vi "main_GB.vi"() -> ()   [LabVIEW 2020]
panel:
  in  "Stop Button":bool
  in  "Setting Tab":enum32{"File", "Setting"}(tab)
  in  "file path (dialog if empty)":path=path "C:/Users/user/Desktop/AutoSampler/AutoSampler _GB/AutoSampler.txt"
  in  "start of read offset (chars.:0)":i32
  in  "max characters/row  (no limit:0)":i32
  out "mark after read (chars.)":i32=403
  in  "number of rows (all:-1)":i32=-1
  out "all rows":string[][](array[string])=[["58"], ["257"], ["0"], ["0"], ["58"], ["257"], ["130"], ["50"], ["58"], ["257"], ["0"], ["50"], ["58"], ["470"], ["0"], ["50"], ["58"], ["470"], ["185"], ["0"], ["58"], ["470"], ["0"], ["0"], ["120"], ["470"], ["0"], ["0"], ["120"], ["470"], ["195"], ["50"], ["120"], ["470"], ["0"], ["50"], ["120"], ["550"], ["0"], ["0"], ["120"], ["550"], ["195"], ["0"], ["120"], ["550"], ["0"], ["0"], ["120"], ["470"], ["0"], ["0"], ["120"], ["470"], ["195"], ["50"], ["120"], ["470"], ["0"], ["50"], ["120"], ["550"], ["0"], ["0"], ["120"], ["550"], ["195"], ["0"], ["120"], ["550"], ["0"], ["0"], ["120"], ["470"], ["0"], ["0"], ["120"], ["470"], ["195"], ["50"], ["120"], ["470"], ["0"], ["50"], ["120"], ["550"], ["0"], ["0"], ["120"], ["550"], ["195"], ["0"], ["120"], ["550"], ["0"], ["0"]]
  in  "format (%.3f)":string="%.3f"
  in  "transpose (no:F)":bool
  in  "type (empty)":string[][](array[string])
  in  "delimiter (Tab)":string="\t"
  out "EOF?":bool
  out "size(s)":i32=96
  in  "Reading Time(S)":dbl=5.0
  out "X, Y, Z, S":i32=3
  out "Index":i32=95
  out "element":string="0"
  out "double precision float":dbl
  out "Current Position(mm)":dbl
  out "Arrived":bool=TRUE
  in  "Occupied Length by Air(mm)":dbl format="%#_13g"
  out "error out":errorcluster={"status"=FALSE, "code"=1073676294, "source"="VISA Read in position_read.vi->main_GB.vi"}
  out "S Connecting":bool=TRUE
  out "Z Connecting":bool=TRUE
  out "Y Connecting":bool=TRUE
  out "X  Connecting":bool=TRUE
  in  "COM Port":refnum<visa-resource-name>="COM3"
  # "Position :"
  # "(set the Occupied length by Air if the target axis is syringe axis)"
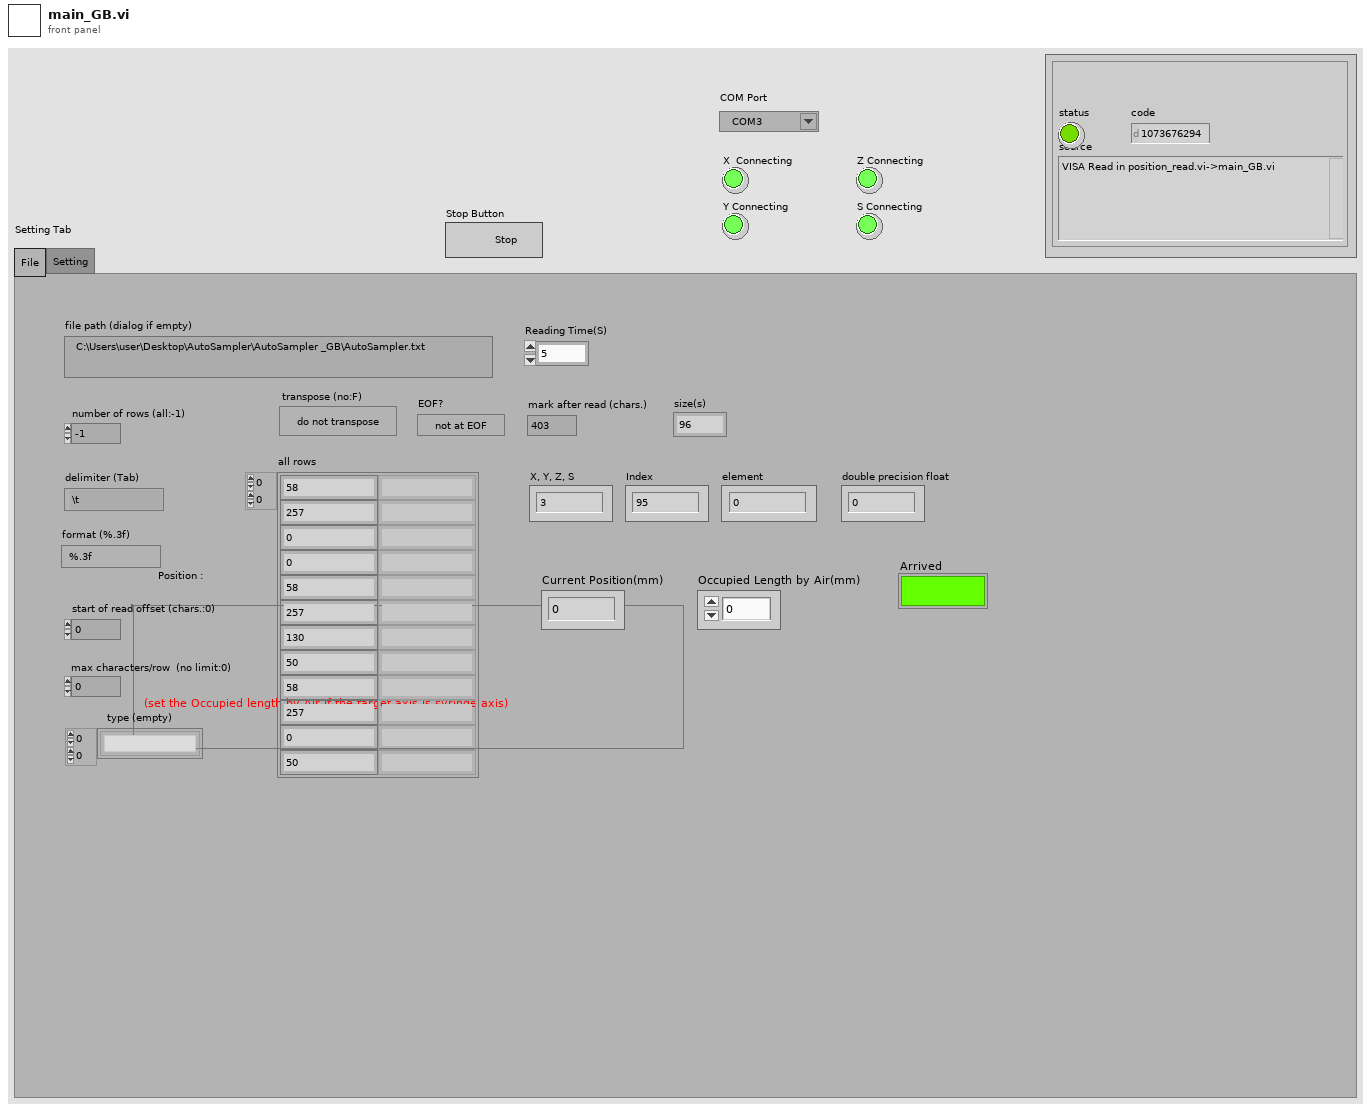
[diagram p1: front panel]
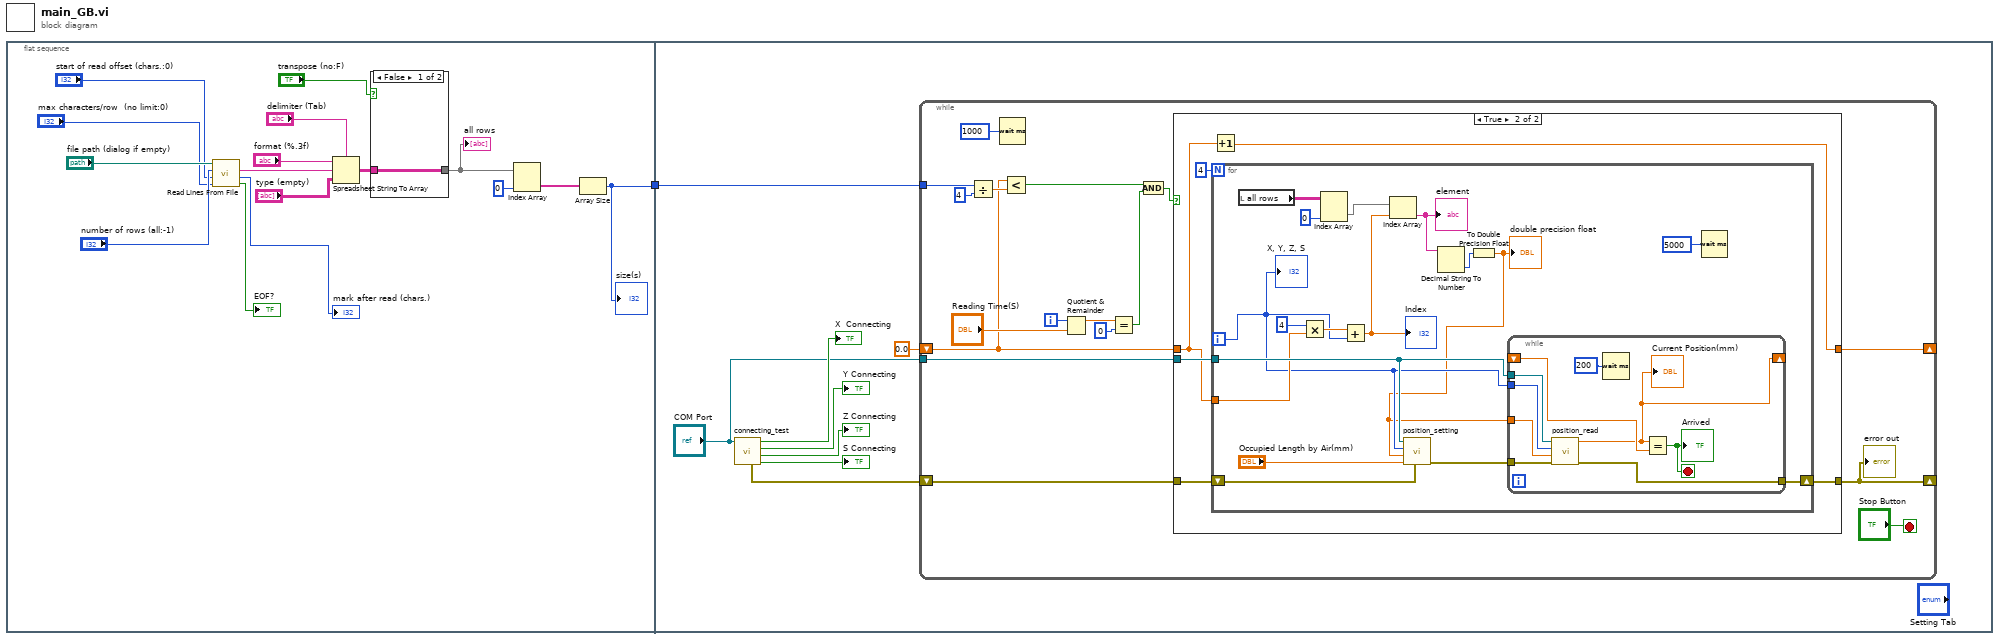
[diagram p0: block diagram]
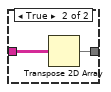
[diagram p2: hidden frame]
diagram:
  n1 = flat-sequence {
    tunnel: [w2] -> w1
    tunnel: w1 -> [w22]
    frame #0 {
      n2 = call <vilib>:"Read Lines From File.vi"("file path (dialog if empty)"="file path (dialog if empty)", "number of lines (all:-1)"="number of rows (all:-1)", "start of read offset (chars.:0)"="start of read offset (chars.:0)", "[max characters per line]  (no limit:0)"="max characters/row  (no limit:0)") -> ("line string"=w13:string, "mark after read (chars.)"=→"mark after read (chars.)":i32, "EOF?"=→"EOF?":bool)  [unwired: 2 in, 1 out]
      n3 = Spreadsheet String To Array(delimiter (Tab)="delimiter (Tab)", format string="format (%.3f)", spreadsheet string=w13, array type (2D Dbl)="type (empty)") -> (array=w11:string[][])
      n4 = case shown="False" "transpose (no:F)" {
        tunnel: [w18 w20] -> w5
        tunnel: w11 -> [w18 w19]
        frame False {
        }
        frame True {
          n5 = Transpose 2D Array(2D array=w19) -> (transposed array=w20:string[][])
        }
      }
      "all rows" <- w5
      n6 = Index Array "Index Array"(array=w5, index (col)=0) -> (element=w3:string[])  [unwired: 1 in]
      n7 = Array Size(array=w3) -> (size(s)=w2:i32)
      "size(s)" <- w2
    }
    frame #1 {
      n8 = call "connecting_test.vi"("VISA resource name"="COM Port") -> ("syringe axis connecting"=→"S Connecting":bool, "Z axis connecting"=→"Z Connecting":bool, "Y axis connecting"=→"Y Connecting":bool, "X axis connecting"=→"X  Connecting":bool, "error out"=w25:errorcluster)  [unwired: 6 in]
      n9 = while {
        shift-right: [w44] -> _
        shift-left: w25 -> [w45]
        tunnel: "COM Port" -> [w41]
        tunnel: w22 -> [w32]
        shift-right: [w30] -> _
        shift-left: 0.0 -> [w29]
        i -> [w38]
        stop <- "Stop Button" stop-if-true
        n10 = Divide(x=w32, y=4) -> (x/y=w35:dbl)
        n11 = Wait (ms)(milliseconds to wait=u32 1000) -> ()  [unwired: 1 out]
        n12 = Less?(x=w29, y=w35) -> (x < y?=w33:bool)
        n13 = Quotient & Remainder(x=w38, y="Reading Time(S)") -> (x-y*floor(x/y)=w37:dbl)  [unwired: 1 out]
        n14 = Equal?(x=w37, y=0) -> (x = y?=w34:bool)
        n15 = And(x=w33, y=w34) -> (x .and. y?=w31:bool)
        n16 = case shown="True" w31 {
          tunnel: w45 -> [w46 w53]
          tunnel: [w46 w52] -> w44
          tunnel: w41 -> [_ w51]
          tunnel: w29 -> [w47 w48]
          tunnel: [w47 w49] -> w30
          frame False {
          }
          frame True {
            n17 = for {
              N: 4 -> [_]
              tunnel: w51 -> [w66]
              shift-right: [w69] -> w52
              shift-left: w53 -> [w70]
              tunnel: w48 -> [w63]
              i -> [w62]
              n18 = local read "all rows"() -> (w60:string[][])
              n19 = Multiply(x=4, y=w63) -> (x*y=w65:dbl)
              n20 = Index Array "Index Array"(array=w60, index (col)=0) -> (element=w61:string[])  [unwired: 1 in]
              n21 = Add(x=w65, y=w62) -> (x+y=w58:dbl)
              "Index" <- w58
              n22 = Index Array(array=w61, index=w58) -> (element=w57:string)
              "element" <- w57
              n23 = Decimal String To Number(string=w57) -> (number=w55:i32)  [unwired: 2 in, 1 out]
              n24 = To Double Precision Float(number=w55) -> (double precision float=w54:dbl)
              "double precision float" <- w54
              n25 = call "position_setting.vi"("error in (no error)"=w70, "Occupied length by Air(mm)"="Occupied Length by Air(mm)", "Distance(mm)"=w54, "Axis"=w62, "Com Port"=w66) -> ("error out"=w68:errorcluster)  [unwired: 6 in]
              n26 = while {
                tunnel: w62 -> [w79]
                tunnel: w54 -> [w78]
                tunnel: [w77] -> w69
                tunnel: w68 -> [w76]
                shift-right: [w74] -> _
                shift-left: _ -> [w75]
                tunnel: w66 -> [w71]
                stop <- w72 stop-if-true
                n27 = call "position_read.vi"("error in (no error)"=w76, "Occupied Length by Air(mm)"=w78, "Axis"=w79, "COM Port"=w71) -> ("error out"=w77:errorcluster, "current position(mm)"=w74:dbl)  [unwired: 6 in]
                "Current Position(mm)" <- w74
                n28 = Wait (ms)(milliseconds to wait=u32 200) -> ()  [unwired: 1 out]
                n29 = Equal?(x=w74, y=w75) -> (x = y?=w72:bool)
                "Arrived" <- w72
              }
              n30 = Wait (ms)(milliseconds to wait=u32 5000) -> ()  [unwired: 1 out]
              "X, Y, Z, S" <- w62
            }
            n31 = Increment(x=w48) -> (x+1=w49:dbl)
          }
        }
        "error out" <- w44
      }
    }
  }
